vi "StatisticsGui.vi"() -> ()   [LabVIEW 2016]
uses:
  Logger/Logger.Stats.Fglb.Result.ctl
  StatisticsGui.Action.ctl
  Logger/Logger.Stats.Fglb.Action.ctl
  <vilib>/Utility/miscctls.llb/LVRowAndColumnTypeDef.ctl
  tools/CitTemplate/citTemplate.errData.ctl
  tools/EventLog/EventLog.EventSource.ctl
  tools/Config/Config.Global.vi
  Global/ApplicationGlobal.vi
  tools/Translator/Translator.Global.vi
  tools/Translator/Translator.Message.ctl
panel:
  out "Graph":cluster{"Graph":dbl[], "Graph":dbl[]}[](graph)
  out "MinTS":timestamp
  out "MaxTS":timestamp
  in  "Table/Graph":bool
  in  "Results.TimeTo":timestamp caption="To" format="%<%x %X>T"
  in  "Results.TimeFrom":timestamp caption="From" format="%<%x %X>T"
  in  "Text Ring":u16(ring) caption="Span"
  out "Results":T1[](array[typedef]) {"Time From" format="%<%X %x>T"; "Time To" format="%<%X %x>T"}
  in  "Values":i32[](listbox) caption="Data"
  out "ValuesRowSelected":i32
  in  "Hider":bool
  in  "StartHere...":bool
  out "_loop":i32(ring)=4
  out "Panel":refnum<vi>
  in  "ResultsAmount":i32=1 caption="Span" min=1 max=100
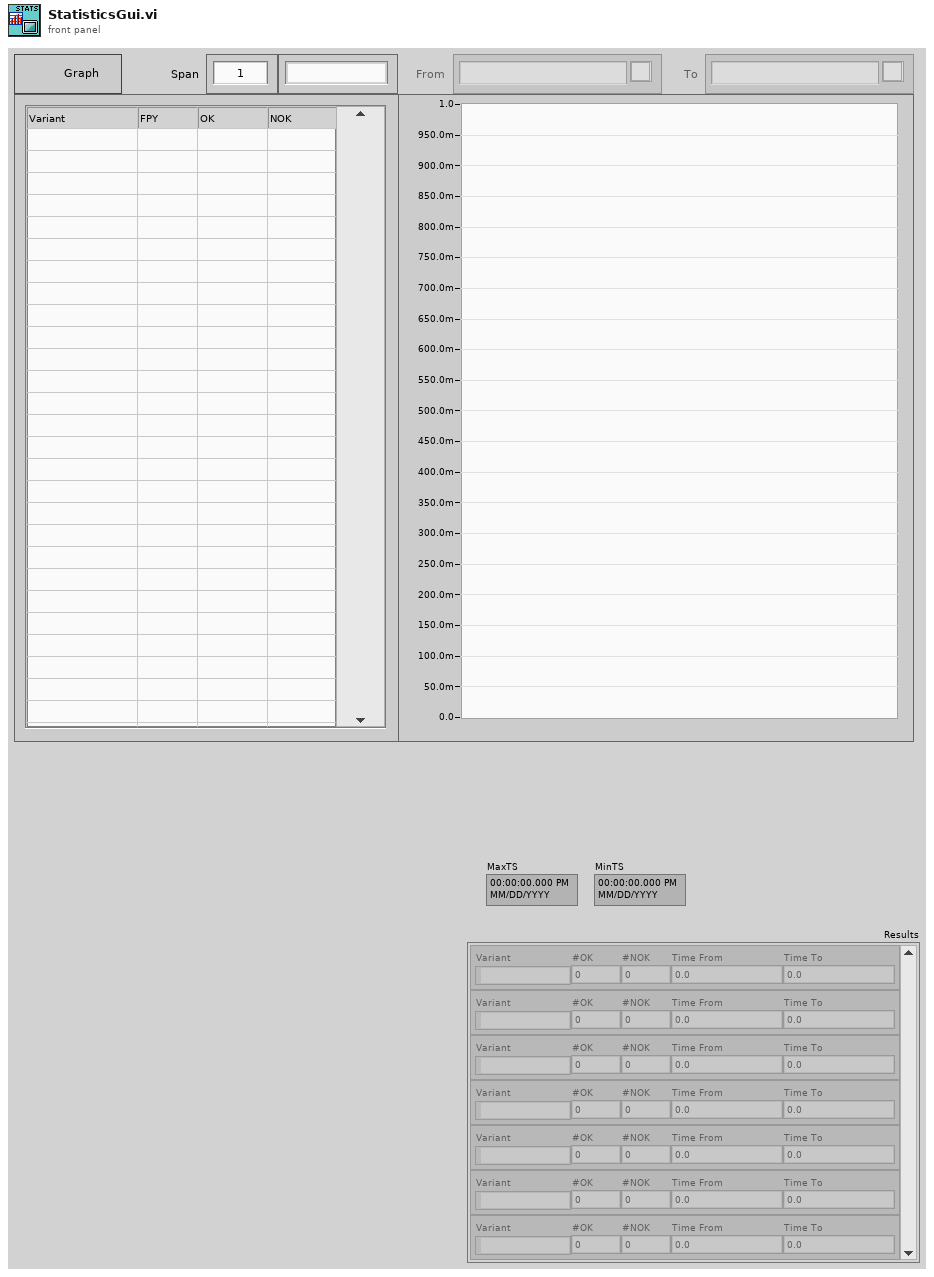
[diagram p1: front panel]
types:
  T1 = typedef "Logger.Stats.Fglb.Result.ctl" = cluster{"Variant":string, "#OK":i32, "#NOK":i32, "Time From":dbl, "Time To":dbl}
  T2 = typedef "StatisticsGui.Action.ctl" = enum32{"idle", "constructor", "destructor", "--- StatisticsGui ---", "new file", "update files", "update table", "update graph", "update time span"}
  T3 = enum8{"Enabled", "Disabled", "Disabled and Grayed Out"}
  T4 = typedef "Logger.Stats.Fglb.Action.ctl" = enum16{"init", "add", "get", "get all"}
  T5 = typedef "LVRowAndColumnTypeDef.ctl" = cluster{"Row":i32, "Column":i32}
  T6 = typedef "citTemplate.errData.ctl" = cluster{"ts":timestamp, "src":T7, "instance":i32, "action":string, "error":errorcluster, "unconfirmed":bool}
  T7 = typedef "EventLog.EventSource.ctl" = enum16{"All", "Gui", "Ref", "File", "Arch", "Seq", "CPX", "DB", "Laser", "Scan.P", "Scan.O"}
  T8 = typedef "citTemplate.notifierHandle.ctl" = refnum<notifier>
  T9 = enum32{"Invalid", "Standard", "Closed", "Hidden", "Minimized", "Maximized"}
  T10 = typedef "LVPoint32TypeDef.ctl" = cluster{"Horizontal":i32, "Vertical":i32}
  T11 = typedef "LVPositionTypeDef.ctl" = cluster{"Left":i32, "Top":i32}
  T12 = typedef "Translator.Message.ctl" = enum16{"-", "Event confirmed", "Log out", "Log in", "Shutdown", "Cancel", "Start", "Begin time", "End time", "Duration", "Service Mode", "Ignore Results", "Serial Format", "On", "Off", "OK", "NOK", "NOK %s", "Home", "Work", "Close", "Open", "In progress...", "Missing", "Empty", "Hardware failure", "Initial", "Default", "Total", "Out of range", "Free disk space is below 1GB - contact technician", "Error %d >> %s", "Error %d >> %s >> %s", "Msg %d >> %s", "Laser msg %d %s", "Laser cmd error %s %d", "Laser cmd failed %s", "Laser cmd warning %s", "Laser disconnected", "Laser status %s", "Laser already started", "Laser job unkonwn %s", "Laser job missing %s", "Laser job select failure %s", "Unable to start laser printing (%s)", "Unable to stop laser printing (%s)", "Laser marking aborted", "Laser marking timeout", "Unable to reset Laser Interlock (%s)", "Unable to trigger Laser. Laser not ready (%s)", "Laser job '%s' coordinates not configured", "Starting %s", "Quitting %s", "Configured", "Initializing", "Quitting", "Loading", "Loaded %d results", "Loaded %d events", "Running", "Stopped", "Summary", "Laser", "Do you want to continue?", "Do you want to delete the configuration?", "The configuration is being used by an order. Unable to delete!", "Press confirm button", "Station is not based. Do you want to exit?", "Station requires changeover. Do you want to run the test?", "Test options are not set as default. Do you want to continue?", "Formatting of WabcoNo is disabled. Do you want to continue?", "Product not detected. Do you want to continue?", "Product scan failed. Do you want to continue?", "Calibration", "Log out?", "System", "All", "IDLE", "Translating...%s", "Not found", "Alarm %s", "Run", "Skip", "Abort", "Repeat", "Please wait...", "Database disconnected", "Database disconnected - changeover disabled!", "Login to database successful", "Login to database failed: %d; %s", "Unable to check the product status of reference %d - database disconnected", "Unable to set the product status of reference %d - database disconnected", "Variant file backup %s", "Read variant (%s)", "Result", "Station armed!", "Station requires changeover!", "Select reference number...", "EMERGENCY BUTTON - press Control button", "EMERGENCY DOOR - press Control button", "Resetting Emergency...", "Unable to reset safety circuit - Emergency Button pressed", "Unable to reset safety circuit - Emergency Side Door open", "Station not based", "Station based", "Station not empty", "Station basing...", "No order", "Press Start to begin new order", "Scanning new order", "Order NOK. Correct or scan again", "Order OK. Press Accept", "Order ready", "Revolver incorrect", "Fork incorrect", "Revolver missing", "Revolver empty", "Container missing", "Offline results", "Offline statistics", "Updating statistics %.1f %%", "DMC Configurator", "Door open", "Close the front door", "Press start button", "Done. Open the front door", "Running...", "Running...%.1f %%", "Pause %s", "Pause %s. NOK container missing", "Pause %s. OK container missing", "Pause %s. Revolver empty", "Pause %s. Revolver missing", "Pause %s. Revolver incorrect", "Pause %s. Fork missing", "Pause %s. Fork incorrect", "Pause %s. Too many failures", "Pause %s. Unloading failure", "Pause %s. One slot is not working", "Pause %s. Part order is done. Empty OK container", "Pause %s. Unable to move product to slot", "Pause %s. Unable to move back product pusher", "Pause %s. Unable to lift product", "Pause %s. Unable to move back product lifter", "Pause %s. Unable to move product arm to Work", "Pause %s. Unable to move product arm to NOK", "Pause %s. Unable to move product arm to OK", "Pause %s. Unable to unsuck the NOK product", "Pause %s. Unable to drop the NOK product", "Pause %s. Product OK missing", "Pause %s. Unable to unsuck the OK product", "Pause %s. Unable to drop the OK product", "Stopping...", "File '%s' is missing", "File '%s' is broken", "File '%s' is running", "Log file started (%s)", "Log file ended (%s)", "Log file stopped (%s)", "Log file ignored (%s)", "Log file exported (%s)", "Log file export failed (%s)", "Wrong serial number in log file", "Wrong reference number in log file", "Test steps are missing", "%s = %.3f", "Process param '%s' not found in DB", "Process param '%s' wrong order", "Process param '%s' value %.3f out of limits (%.3f; %.3f)", "Step%d param '%s' not found in DB", "Step%d param '%s' wrong order", "Step%d param '%s' value %.3f out of limits (%.3f; %.3f)", "Step%d EV '%s' not found in DB", "Step%d EV '%s' wrong order", "\"%s\" not found in DB", "\"%s\" wrong order", "\"%s\" value %.3f out of limits (%.3f; %.3f)", "\"%s\" not found in software", "Process init (%s)", "Process started", "Process restarted", "Process run", "Process done", "Process done - remove OK container", "Process aborted", "Process aborted at work", "Process aborted at home", "Process error", "Process error at home", "Process error at work", "Process close", "Process pause", "Process continue", "Process door open", "Process door close", "Process pause at slot %s due to %s", "Select plate from the order to process", "Do you want to start the process?", "Do you want to continue the process?", "There is unfinished order. Do you want to put the new order?", "Product %s %d OK", "Product %s %d NOK", "Unable to unload the slot %s. Product missing in the slot", "Unable to unload the slot %s. Product already in the arm", "Unable to accept the product as OK. Product missing in slot %s", "Unable to accept the product as OK. Product could not drop into the container at slot %s", "Unable to accept the product as NOK. Product could not drop into the container at slot %s", "Scan failed. Error %s", "Scan failed. Scanner disconnected", "Scan failed. Wrong Wabco number %d, limit (%d,%d)", "Scan failed. Wrong serial number %d, limit (%d,%d)", "Scan failed. Wrong date %d, limit (%d,%d)", "Scan failed. Wrong product wabco number %d (expected %d)", "Scan failed. Wrong product serial number %d (expected > 0)", "Scan OK %s", "Scan failed. Unable to determine table position (%s)", "Scan failed. Timeout", "Tune failed. Scanner disconnected", "Tune failed. Timeout", "%s = %d", "%s = %d->%d", "Unable to set %s = %.2f - Air Pressure Inside off", "Unable to set digital output '%s' = %d", "Unable to activate air pressure inside - timeout", "Unable to activate air pressure inside - aborted", "Unable to switch on Air Main Valve - Air Pressure Inlet off", "Unable to switch on Air Main Valve - Door open", "Unable to switch off Air Main Valve - timeout", "Unable to switch off Air Main Valve - aborted", "Unable to rotate Table - timeout", "Unable to rotate Table - aborted", "Unable to rotate Table - Product Move not in Home position", "Unable to rotate Table - Air Pressure Inside off", "Unable to rotate Table - Product Lift A not in Home position", "Unable to rotate Table - Product Lift B not in Home position", "Unable to rotate Table - unlock before movement timeout", "Unable to rotate Table - lock after movement timeout", "Unable to move Table Lock to %s position - timeout", "Unable to move Table Lock to %s position - aborted", "Unable to move Table Lock to %s position - Air Pressure Inside off", "Unable to move Table Lock to %s position - Table not in position", "Unable to move Product Lift A to %s position - timeout", "Unable to move Product Lift B to %s position - timeout", "Unable to move Product Lift A to %s position - aborted", "Unable to move Product Lift B to %s position - aborted", "Unable to move Product Lift A to %s position - Air Pressure Inside off", "Unable to move Product Lift B to %s position - Air Pressure Inside off", "Unable to move Product Lift A to %s position - Table not locked", "Unable to move Product Lift B to %s position - Table not locked", "Unable to move Product Lift A to %s position - Product Arm not in Work position", "Unable to move Product Lift B to %s position - Product Arm not in Work position", "Unable to set Product Suction Gripper %s to %s - timeout", "Unable to set Product Suction Gripper %s to %s - aborted", "Unable to set Product Suction Gripper %s to %s - Air Pressure Inside off", "Unable to set Product Suction Gripper %s to %s - Table slot unkown", "Unable to move Product Arm to %s position - timeout", "Unable to move Product Arm to %s position - aborted", "Unable to move Product Arm to %s position - Air Pressure Inside off", "Unable to move Product Arm to %s position - Product Lift A not in Home position", "Unable to move Product Arm to %s position - Product Lift B not in Home position", "Unable to move Product to %s position - timeout", "Unable to move Product to %s position - aborted", "Unable to move Product to %s position - Air Pressure Inside off", "Unable to move Product to %s position - Table not in position"}
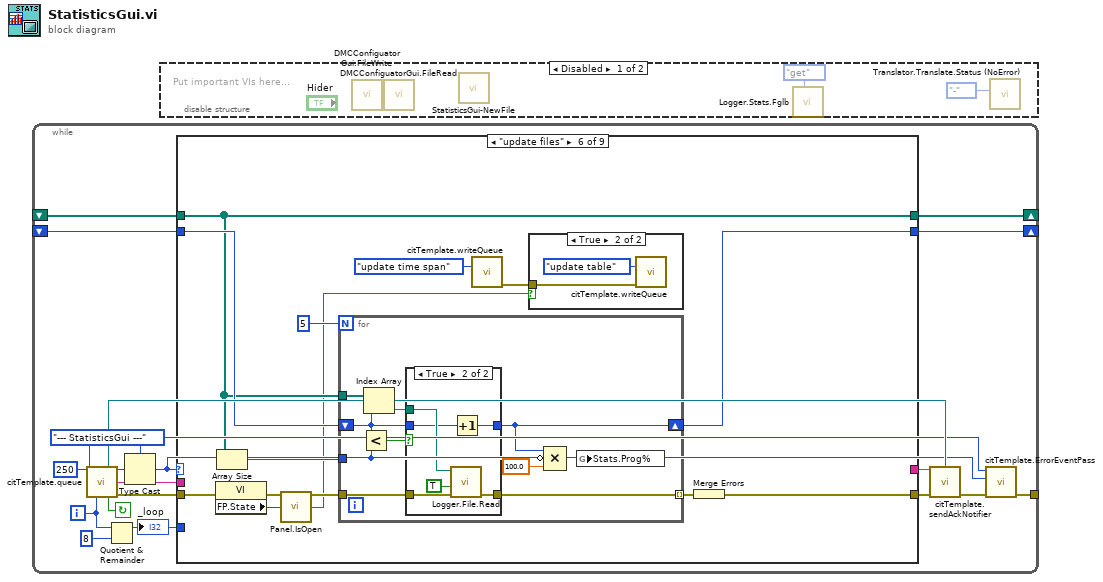
[diagram p0: block diagram]
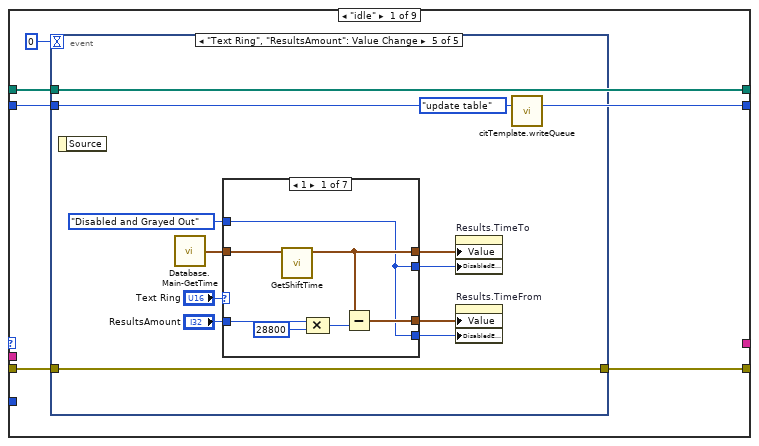
[diagram p2: hidden frame]
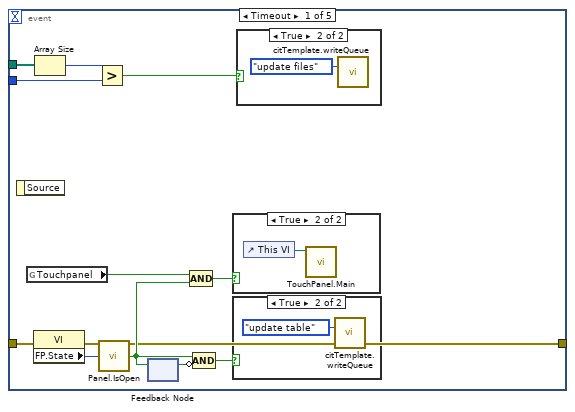
[diagram p3: hidden frame]
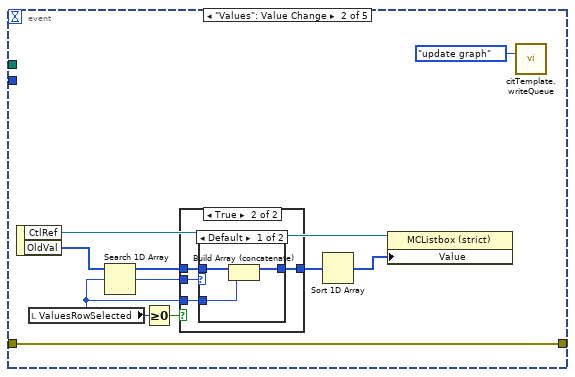
[diagram p7: hidden frame]
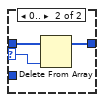
[diagram p9: hidden frame]
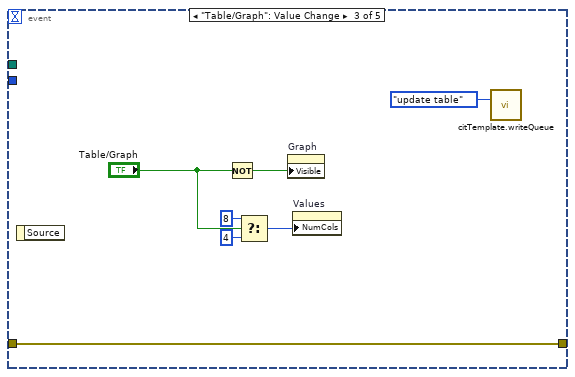
[diagram p10: hidden frame]
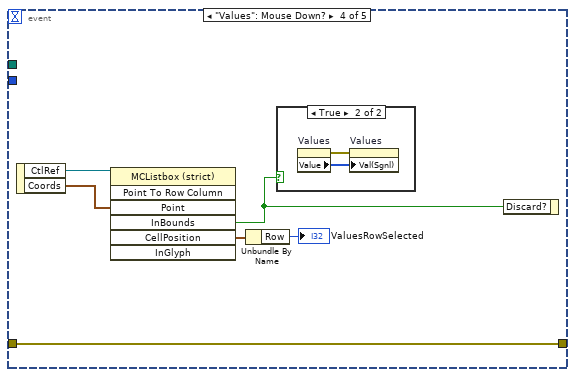
[diagram p11: hidden frame]
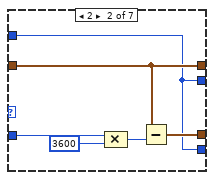
[diagram p13: hidden frame]
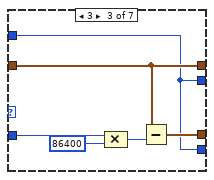
[diagram p14: hidden frame]
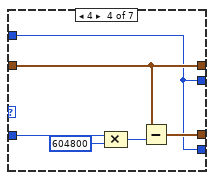
[diagram p15: hidden frame]
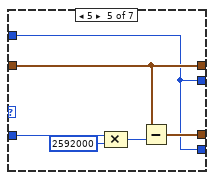
[diagram p16: hidden frame]
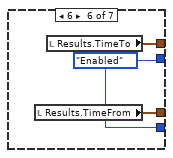
[diagram p17: hidden frame]
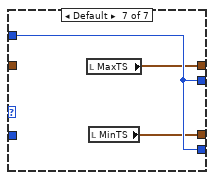
[diagram p18: hidden frame]
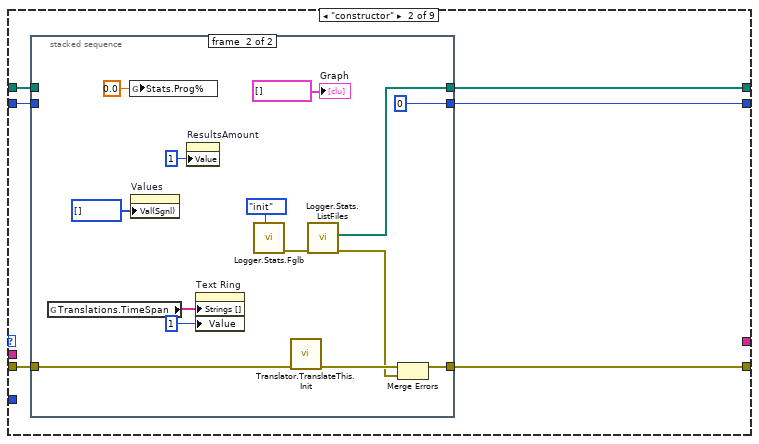
[diagram p19: hidden frame]
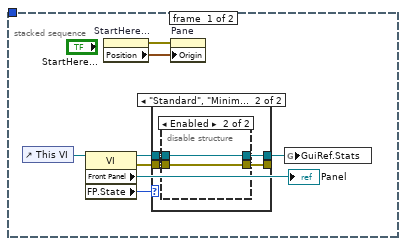
[diagram p20: hidden frame]
diagram:
  n1 = while {
    tunnel: [w7] -> _
    shift-right: [w4] -> _
    shift-left: _ -> [w3]
    shift-right: [w2] -> _
    shift-left: _ -> [w1]
    i -> [w9]
    stop <- w15 continue-if-true
    w12 = StatisticsGui.Action."--- StatisticsGui ---" ("Action")
    n2 = call "citTemplate.queue.vi"("ms timeout (250 ms)"=250, "event enum"=w12, "iteration (-1)"=w9) -> ("notifierHandle out"=w14:T8, "event out"=w18:u32, "(flatten) data out"=w17:string, "continue"=w15:bool, "error out"=w16:errorcluster)  [unwired: 2 in, 6 out]
    n3 = Quotient & Remainder(x=w9, y=8) -> (x-y*floor(x/y)=w5:i32)  [unwired: 1 out]
    "_loop" <- w5
    n4 = Type Cast(type=w12, x=w18) -> (*(type *) &x=w8:T2)
    n5 = case shown="\"update files\"" w8 {
      tunnel: w17 -> [_ _ _ w184 w193 _ _ _ _]
      tunnel: w16 -> [w23 w125 w163 w182 w192 w199 w230 w295 w319]
      tunnel: [_ _ _ "" _ _ _ _ _] -> w13
      tunnel: [w21 w126 w164 w183 w186 w196 w229 w296 w318] -> w11
      tunnel: w5 -> [_ _ _ _ _ _ _ _ _]
      tunnel: [w20 w124 w162 w178 w189 w203 w228 w294 w317] -> w4
      tunnel: w3 -> [w20 w123 w162 w178 w190 w203 w228 w294 w317]
      tunnel: [w19 w122 w161 w177 w191 w201 w227 w293 w316] -> w2
      tunnel: w1 -> [w19 w121 w161 w177 w191 w204 w227 w293 w316]
      frame "idle" {
        n6 = event shown="[4] \"Text Ring\", \"ResultsAmount\": Value Change" {
          selector: _ -> [_ _ _ _ _]
          dyn-events: _ -> [_ _ _ _ _]
          timeout: 0 -> [_ _ _ _ _]
          tunnel: w23 -> [w35 w45 w60 w66 w81]
          tunnel: [w24 w45 w60 w66 w81] -> w21
          tunnel: w20 -> [w28 _ _ _ _]
          tunnel: w19 -> [w26 _ _ _ _]
          event Timeout {
            n7 = event-data() -> ()  [unwired: 1 in, 1 out]
            n8 = global read "Config.Global.vi" "Touchpanel"() -> (w32:bool)
            n9 = property class="VI"(error in=w35) -> (error out=w24:errorcluster, "FP.State"=w33:T9)  [unwired: 1 in, 1 out]
            n10 = Array Size(array=w28) -> (size(s)=w25:i32)
            n11 = Greater?(x=w25, y=w26) -> (0:w27:bool)
            n12 = call "Panel.IsOpen.vi"("FP State"=w33) -> ("Open?"=w29:bool)
            n13 = feedback-in #1(w29) -> ()
            n14 = feedback #1() -> (w34:bool)  [unwired: 1 in]
            n15 = Compound Arithmetic op=AND(w32, w29) -> (w31:bool)
            n16 = Compound Arithmetic op=AND(w29, invert w34) -> (w30:bool)
            n17 = case shown="True" w31 {
              frame False {
              }
              frame True {
                n18 = control-ref of="This VI"() -> (w38:refnum<vi>)
                n19 = call "TouchPanel.Main.vi"("VI ref"=w38) -> ()  [unwired: 8 in, 3 out]
              }
            }
            n20 = case shown="True" w30 {
              frame False {
              }
              frame True {
                n21 = call "citTemplate.writeQueue.vi"("event in (if not connected:all statemachine with data event)"=StatisticsGui.Action."update table" ("Action")) -> ()  [unwired: 14 in, 1 out]
              }
            }
            n22 = case shown="True" w27 {
              frame False {
              }
              frame True {
                n23 = call "citTemplate.writeQueue.vi"("event in (if not connected:all statemachine with data event)"=StatisticsGui.Action."update files" ("Action")) -> ()  [unwired: 14 in, 1 out]
              }
            }
          }
          event "Values": Value Change {
            n24 = event-data() -> ("CtlRef"=w47:refnum<vi>, "OldVal"=w44:i32[])  [unwired: 1 in]
            n25 = local read "ValuesRowSelected"() -> (w41:i32)
            n26 = Search 1D Array(1D array=w44, element=w41) -> (index of element=w46:i32)  [unwired: 1 in]
            n27 = Greater Or Equal To 0?(x=w41) -> (x >= 0?=w43:bool)
            n28 = case shown="True" w43 {
              tunnel: w46 -> [_ w52]
              tunnel: w44 -> [w48 w51]
              tunnel: [w48 w50] -> w42
              tunnel: w41 -> [_ w49]
              frame False {
              }
              frame True {
                n29 = case shown="Default" w52 {
                  selector: w52 -> [_ w57]
                  tunnel: w51 -> [w55 w58]
                  tunnel: [w54 w56] -> w50
                  tunnel: w49 -> [w53 _]
                  frame Default {
                    n30 = Build Array (concatenate)(w55, w53) -> (w54:i32[])
                  }
                  frame 0.. {
                    n31 = Delete From Array(array=w58, index=w57) -> (array with subset deleted=w56:i32[])  [unwired: 1 in, 1 out]
                  }
                }
              }
            }
            n32 = Sort 1D Array(array=w42) -> (sorted array=w39:i32[])
            n33 = property class="MCListbox (strict)"(reference=w47, "Value"=w39) -> ()  [unwired: 1 in, 2 out]
            n34 = call "citTemplate.writeQueue.vi"("event in (if not connected:all statemachine with data event)"=StatisticsGui.Action."update graph" ("Action")) -> ()  [unwired: 14 in, 1 out]
          }
          event "Table/Graph": Value Change {
            n35 = event-data() -> ()  [unwired: 1 in, 1 out]
            n36 = Not(x="Table/Graph") -> (.not. x?=w65:bool)
            n37 = Select(t=u32 8 ("Number of Columns"), s="Table/Graph", f=u32 4 ("Number of Columns")) -> (s? t:f=w62:u32)
            n38 = property on="Graph" class="XYGraph (strict)"("Visible"=w65) -> ()  [unwired: 2 in, 2 out]
            n39 = property on="Values" class="MCListbox (strict)"("NumCols"=w62) -> ()  [unwired: 2 in, 2 out]
            n40 = call "citTemplate.writeQueue.vi"("event in (if not connected:all statemachine with data event)"=StatisticsGui.Action."update table" ("Action")) -> ()  [unwired: 14 in, 1 out]
          }
          event "Values": Mouse Down? {
            n41 = event-data() -> ("CtlRef"=w71:refnum<vi>, "Coords"=w70:T10)  [unwired: 1 in]
            n42 = invoke class="MCListbox (strict)" method="Point To Row Column"(reference=w71, "Point"=w70) -> ("InBounds"=w67:bool, "CellPosition"=w69:T5)  [unwired: 5 in, 5 out]
            n43 = Unbundle By Name(w69) -> ("Row"=→"ValuesRowSelected":i32)
            n44 = case shown="True" w67 {
              frame False {
              }
              frame True {
                n45 = property on="Values" class="MCListbox (strict)"() -> (error out=w73:errorcluster, "Value"=w72:i32[])  [unwired: 2 in, 1 out]
                n46 = property on="Values" class="MCListbox (strict)"(error in=w73, "Val(Sgnl)"=w72) -> ()  [unwired: 1 in, 2 out]
              }
            }
            n47 = event-data("Discard?"=w67) -> ()  [unwired: 1 in, 1 out]
          }
          event "Text Ring", "ResultsAmount": Value Change {
            n48 = event-data() -> ()  [unwired: 1 in, 1 out]
            n49 = call "Database.Main-GetTime.vi"() -> ("TS"=w74:timestamp)  [unwired: 1 in]
            n50 = case shown="1" "Text Ring" {
              tunnel: [w88 w95 w101 w107 w113 w117 w119] -> w80
              tunnel: w74 -> [w89 w95 w101 w107 w113 _ _]
              tunnel: [w85 w96 w102 w108 w114 w116 w118] -> w79
              tunnel: "ResultsAmount" -> [w87 w94 w100 w106 w112 _ _]
              tunnel: [w84 w91 w97 w103 w109 w115 w120] -> w78
              tunnel: [w84 w91 w97 w103 w109 w115 w120] -> w77
              tunnel: T3."Disabled and Grayed Out" ("Disabled") -> [w84 w91 w97 w103 w109 _ w120]
              frame 1 {
                n51 = call "GetShiftTime.vi"("Time"=w89) -> ("Shift End Time"=w88:timestamp)  [unwired: 7 in, 3 out]
                n52 = Compound Arithmetic op=MULTIPLY(w87, 28800) -> (w86:i32)
                n53 = Subtract(x=w88, y=w86) -> (x-y=w85:timestamp)
              }
              frame 2 {
                n54 = Compound Arithmetic op=MULTIPLY(w94, 3600) -> (w93:i32)
                n55 = Subtract(x=w95, y=w93) -> (x-y=w96:timestamp)
              }
              frame 3 {
                n56 = Compound Arithmetic op=MULTIPLY(w100, 86400) -> (w99:i32)
                n57 = Subtract(x=w101, y=w99) -> (x-y=w102:timestamp)
              }
              frame 4 {
                n58 = Compound Arithmetic op=MULTIPLY(w106, 604800) -> (w105:i32)
                n59 = Subtract(x=w107, y=w105) -> (x-y=w108:timestamp)
              }
              frame 5 {
                n60 = Compound Arithmetic op=MULTIPLY(w112, 2592000) -> (w111:i32)
                n61 = Subtract(x=w113, y=w111) -> (x-y=w114:timestamp)
              }
              frame 6 {
                w115 = T3."Enabled" ("Disabled")
                n62 = local read "Results.TimeFrom"() -> (w116:timestamp)
                n63 = local read "Results.TimeTo"() -> (w117:timestamp)
              }
              frame Default {
                n64 = local read "MaxTS"() -> (w119:timestamp)
                n65 = local read "MinTS"() -> (w118:timestamp)
              }
            }
            n66 = property on="Results.TimeTo" class="AbsTime (strict)"("Value"=w80, "DisabledEnum"=w77) -> ()  [unwired: 2 in, 2 out]
            n67 = property on="Results.TimeFrom" class="AbsTime (strict)"("Value"=w79, "DisabledEnum"=w78) -> ()  [unwired: 2 in, 2 out]
            n68 = call "citTemplate.writeQueue.vi"("event in (if not connected:all statemachine with data event)"=StatisticsGui.Action."update table" ("Action")) -> ()  [unwired: 14 in, 1 out]
          }
        }
      }
      frame "constructor" {
        n69 = stacked-sequence {
          tunnel: [_ w152] -> w126
          tunnel: w125 -> [_ w160]
          tunnel: [_ w158] -> w124
          tunnel: w123 -> [_ _]
          tunnel: [_ 0] -> w122
          tunnel: w121 -> [_ _]
          frame #0 {
            n70 = control-ref of="This VI"() -> (w132:refnum<vi>)
            n71 = property class="VI"(reference=w132) -> (reference out=w131:refnum<vi>, error out=w130:errorcluster, "Front Panel"=→"Panel":refnum<vi>, "FP.State"=w129:T9)  [unwired: 1 in]
            n72 = property on="StartHere..." class="Bool (strict)"() -> (error out=w134:errorcluster, "Position"=w133:T11)  [unwired: 2 in, 1 out]
            n73 = case shown="\"Standard\", \"Minimized\", \"Maximized\"" w129 {
              tunnel: w131 -> [w136 w140]
              tunnel: w130 -> [w135 w139]
              tunnel: [w136 w138] -> w128
              tunnel: [w135 w137] -> _
              frame Default {
              }
              frame "Standard", "Minimized", "Maximized" {
                n74 = disable-structure shown="Enabled" {
                  disable-tunnel: w140 -> [w144 w146]
                  disable-tunnel: w139 -> [w143 w145]
                  disable-tunnel: [w142 w146] -> w138
                  disable-tunnel: [w141 w145] -> w137
                  frame Disabled {
                    n75 = invoke class="VI" method="FP.Close"(reference=w144, error in=w143) -> (reference out=w142:refnum<vi>, error out=w141:errorcluster)  [unwired: 1 in, 1 out]
                  }
                  frame Enabled {
                  }
                }
              }
            }
            n76 = property on="Pane" class="Pane"(error in=w134, "Origin"=w133) -> ()  [unwired: 1 in, 2 out]
            n77 = global write "ApplicationGlobal.vi" "GuiRef.Stats"(w128) -> ()
          }
          frame #1 {
            n78 = global read "Translator.Global.vi" "Translations.TimeSpan"() -> (w149:string[])
            n79 = global write "ApplicationGlobal.vi" "Stats.Prog%"(0.0 ("Stats.Prog%")) -> ()
            n80 = property on="Values" class="MCListbox (strict)"("Val(Sgnl)"=i32[] [] ("Value (Signaling)")) -> ()  [unwired: 2 in, 2 out]
            n81 = property on="ResultsAmount" class="DigNum (strict)"("Value"=1 ("ResultsAmount")) -> ()  [unwired: 2 in, 2 out]
            n82 = property on="Text Ring" class="Ring (strict)"("Strings []"=w149, "Value"=1) -> ()  [unwired: 2 in, 2 out]
            n83 = call "Logger.Stats.Fglb.vi"("Action (get)"=Logger.Stats.Fglb.Action."init" ("Action")) -> ("error out"=w154:errorcluster)  [unwired: 9 in, 1 out]
            n84 = call "Translator.TranslateThis.Init.vi"("error in"=w160) -> ("error out"=w153:errorcluster)  [unwired: 10 in]
            n85 = call "Logger.Stats.ListFiles.vi"("error in (no error)"=w154) -> ("error out"=w151:errorcluster, "Files"=w158:path[])  [unwired: 9 in]
            n86 = Merge Errors(w153, w151) -> (w152:errorcluster)
            "Graph" <- cluster{"Graph":dbl[], "Graph":dbl[]}[] [] ("Graph")
          }
        }
      }
      frame "destructor" {
        n87 = stacked-sequence {
          tunnel: [_ w176] -> w164
          tunnel: w163 -> [_ w175]
          frame #0 {
            n88 = local read "Panel"() -> (w173:refnum<vi>)
            n89 = property class="Pnl"(reference=w173, "DeferPanUpdts"=FALSE ("Defer Panel Updates")) -> (reference out=w171:refnum<vi>, error out=w170:errorcluster)  [unwired: 1 in]
            n90 = Close Reference(reference=w171, error in (no error)=w170) -> ()  [unwired: 1 out]
            n91 = property on="Values" class="MCListbox (strict)"("ItemNames"=string[][] [] ("Item Names"), "ActiveCell"=T5 {"Row"=-2, "Column"=-2} ("Active Cell:Active Cell"), "CellBG"=u32 16448250, "ActiveCell"=T5 {"Row"=-1, "Column"=-2} ("Active Cell:Active Cell"), "CellBG"=u32 13816530) -> ()  [unwired: 2 in, 2 out]
          }
          frame #1 {
            n92 = property on="Text Ring" class="Ring (strict)"("Strings []"=string[] []) -> ()  [unwired: 2 in, 2 out]
            n93 = call "Translator.TranslateThis.Exit.vi"("error in"=w175) -> ("error out"=w176:errorcluster)  [unwired: 10 in]
          }
        }
      }
      frame "--- StatisticsGui ---" {
        n94 = Unflatten From String(type=T6 {"ts"=timestamp(0 s since 1904-01-01), "src"=enum."All", "instance"=0, "action"="", "error"={"status"=FALSE, "code"=0, "source"=""}, "unconfirmed"=FALSE} ("ErrData"), binary string=w184, error in (no error)=w182) -> (value=w180:T6)  [unwired: 4 out]
        n95 = Unbundle By Name(w180) -> ("error"=w179:errorcluster)
        n96 = call <vilib>:"Clear Errors.vi"("error in (no error)"=w179) -> ("error out"=w183:errorcluster)  [unwired: 5 in, 1 out]
      }
      frame "new file" {
        n97 = Unflatten From String(type=path "", binary string=w193, error in (no error)=w192) -> (value=w187:path, error out=w186:errorcluster)  [unwired: 3 out]
        n98 = Build Array (concatenate)(w190, w187) -> (w189:path[])
      }
      frame "update files" {
        n99 = property class="VI"(error in=w199) -> (error out=w198:errorcluster, "FP.State"=w200:T9)  [unwired: 1 in, 1 out]
        n100 = Array Size(array=w203) -> (size(s)=w202:i32)
        n101 = call "Panel.IsOpen.vi"("FP State"=w200) -> ("Open?"=w197:bool)
        n102 = for {
          N: 5 -> [_]
          tunnel: w203 -> [w216]
          shift-right: [w209] -> w201
          shift-left: w204 -> [w213]
          tunnel: w202 -> [w210]
          tunnel: w198 -> [w218]
          tunnel: [w217] -> w206 mode=indexing
          n103 = Less?(x=w213, y=w210) -> (x < y?=w214:bool)
          n104 = Index Array(array=w216, index=w213) -> (element=w215:path)
          n105 = case shown="True" w214 {
            tunnel: w218 -> [w220 w225]
            tunnel: [w220 w224] -> w217
            tunnel: [w219 w223] -> w209
            tunnel: w215 -> [_ w222]
            tunnel: w213 -> [w219 w221]
            frame False {
            }
            frame True {
              n106 = call "Logger.File.Read.vi"("error in (no error)"=w225, "Update Stats (F)"=TRUE, "file path"=w222) -> ("error out"=w224:errorcluster)  [unwired: 5 in, 3 out]
              n107 = Increment(x=w221) -> (x+1=w223:i32)
            }
          }
          n108 = Compound Arithmetic op=MULTIPLY(w209, invert w210, 100.0 ("value")) -> (w211:dbl)
          n109 = global write "ApplicationGlobal.vi" "Stats.Prog%"(w211) -> ()
        }
        n110 = call "citTemplate.writeQueue.vi"("event in (if not connected:all statemachine with data event)"=StatisticsGui.Action."update time span" ("Action")) -> ("error out"=w194:errorcluster)  [unwired: 14 in]
        n111 = case shown="True" w197 {
          tunnel: w194 -> [_ w207]
          frame False {
          }
          frame True {
            n112 = call "citTemplate.writeQueue.vi"("event in (if not connected:all statemachine with data event)"=StatisticsGui.Action."update table" ("Action"), "error in (no error)"=w207) -> ()  [unwired: 13 in, 1 out]
          }
        }
        n113 = Merge Errors(w206) -> (w196:errorcluster)
      }
      frame "update table" {
        n114 = stacked-sequence {
          seq-local: [_ w234 _ _ _] -> [_ _ _ w283 _]
          tunnel: w230 -> [_ _ w253 _ _]
          tunnel: [_ _ w252 _ _] -> w229
          frame #0 {
            n115 = local read "Panel"() -> (w231:refnum<vi>)
            n116 = property class="Pnl"(reference=w231, "DeferPanUpdts"=TRUE ("Defer Panel Updates")) -> ()  [unwired: 1 in, 2 out]
          }
          frame #1 {
            n117 = property on="Values" class="MCListbox (strict)"() -> (error out=w233:errorcluster, "ItemNames"=w236:string[][], "Value"=w235:i32[])  [unwired: 2 in, 1 out]
            n118 = for {
              tunnel: w236 -> [w244]
              tunnel: w235 -> [w243] mode=indexing
              tunnel: [w242] -> w234 mode=indexing
              n119 = Index Array(array=w244, index (row)=w243, index (col)=0 ("disabled index (col)")) -> (element=w242:string)
            }
            n120 = property on="Values" class="MCListbox (strict)"(error in=w233, "ActiveCell"=T5 {"Row"=-2, "Column"=-2} ("Active Cell:Active Cell"), "CellBG"=u32 16448250, "ActiveCell"=T5 {"Row"=-1, "Column"=-2} ("Active Cell:Active Cell"), "CellBG"=u32 13816530) -> ()  [unwired: 1 in, 2 out]
          }
          frame #2 {
            n121 = To Double Precision Float(number="Results.TimeFrom") -> (double precision float=w246:dbl)
            n122 = To Double Precision Float(number="Results.TimeTo") -> (double precision float=w248:dbl)
            n123 = call "Logger.Stats.Fglb.vi"("Time To"=w248, "Time From"=w246, "Action (get)"=Logger.Stats.Fglb.Action."get" ("Action"), "error in (no error)"=w253) -> ("error out"=w252:errorcluster, "Results"=w250:T1[])  [unwired: 6 in]
            "Results" <- w250
            n124 = call "citTemplate.writeQueue.vi"("event in (if not connected:all statemachine with data event)"=StatisticsGui.Action."update graph" ("Action")) -> ()  [unwired: 14 in, 1 out]
            n125 = for {
              tunnel: w250 -> [w269] mode=indexing
              tunnel: [w281] -> w251 mode=indexing
              i -> [w264]
              w278 = "%Y-%m-%d %H:%M:%S" ("time format string (%c)")
              n126 = Unbundle(w269) -> ("Variant"=w257:string, "#OK"=w267:i32, "#NOK"=w268:i32, "Time From"=w256:dbl, "Time To"=w255:dbl)
              n127 = Compound Arithmetic op=ADD(w267, w268) -> (w261:i32)
              n128 = Bundle(w264, "precision (6)"=i16 1) -> (w262:cluster{i32, "precision (6)":i16})  [unwired: 1 in]
              n129 = call "Int2Str.vi"("Numeric"=w267) -> ("string"=w280:string)
              n130 = Compound Arithmetic op=MULTIPLY(100.0 ("value"), w267, invert w261) -> (w259:dbl)
              n131 = call "Int2Str.vi"("Numeric"=w268) -> ("string"=w279:string)
              n132 = call "DblNaN2Str.vi"("Numeric"=w259, "precision (6)"=i16 2) -> ("string"=w266:string)
              n133 = Format Date/Time String(time format string (%c)=w278, seconds (now)=w256) -> (date/time string=w277:string)  [unwired: 1 in]
              n134 = Format Date/Time String(time format string (%c)=w278, seconds (now)=w255) -> (date/time string=w275:string)  [unwired: 1 in]
              n135 = Greater Than 0?(x=w256) -> (x > 0?=w276:bool)
              n136 = Greater Than 0?(x=w255) -> (x > 0?=w274:bool)
              n137 = call "StatisticsGui.FPYcolor.vi"("result"=w259) -> ("Color"=w258:u32)
              n138 = Select(t=w277, s=w276, f="") -> (s? t:f=w271:string)
              n139 = Select(t=w275, s=w274, f="") -> (s? t:f=w270:string)
              n140 = property on="Values" class="MCListbox (strict)"("ActiveCell"=w262, "CellBG"=w258) -> ()  [unwired: 2 in, 2 out]
              n141 = Build Array(w257, w266, w280, w279, w271, w270) -> (w281:string[])
            }
            n142 = property on="Values" class="MCListbox (strict)"("ItemNames"=w251) -> ()  [unwired: 2 in, 2 out]
          }
          frame #3 {
            n143 = property on="Values" class="MCListbox (strict)" props=["ItemNames", "Value"]() -> ("ItemNames"=w286:string[][])  [unwired: 2 in, 3 out]
            n144 = Index Array(array=w286, index (col)=0 ("disabled index (col)")) -> (element=w284:string[])  [unwired: 1 in]
            n145 = for {
              tunnel: w284 -> [w290]
              tunnel: w283 -> [w289] mode=indexing
              tunnel: [w288] -> w282 mode=indexing if=w287
              n146 = Search 1D Array(1D array=w290, element=w289) -> (index of element=w288:i32)  [unwired: 1 in]
              n147 = Greater Or Equal To 0?(x=w288) -> (x >= 0?=w287:bool)
            }
            n148 = property on="Values" class="MCListbox (strict)"("Value"=w282) -> ()  [unwired: 2 in, 2 out]
          }
          frame #4 {
            n149 = local read "Panel"() -> (w291:refnum<vi>)
            n150 = property class="Pnl"(reference=w291, "DeferPanUpdts"=FALSE ("Defer Panel Updates")) -> ()  [unwired: 1 in, 2 out]
          }
        }
      }
      frame "update graph" {
        n151 = stacked-sequence {
          tunnel: [_ w302 _] -> w296
          tunnel: w295 -> [_ w301 _]
          frame #0 {
            n152 = local read "Panel"() -> (w297:refnum<vi>)
            n153 = property class="Pnl"(reference=w297, "DeferPanUpdts"=TRUE ("Defer Panel Updates")) -> ()  [unwired: 1 in, 2 out]
          }
          frame #1 {
            n154 = control-ref of="Graph"() -> (w299:refnum<vi>)
            n155 = local read "Results"() -> (w303:T1[])
            n156 = call "Logger.Stats.UpdateGraph.vi"("error in (no error)"=w301, "Selection"="Values", "Results"=w303, "Graph"=w299) -> ("error out"=w302:errorcluster)  [unwired: 7 in]
          }
          frame #2 {
            n157 = local read "Panel"() -> (w304:refnum<vi>)
            n158 = property class="Pnl"(reference=w304, "DeferPanUpdts"=FALSE ("Defer Panel Updates")) -> ()  [unwired: 1 in, 2 out]
          }
        }
      }
      frame "update time span" {
        n159 = call "Logger.Stats.Fglb.vi"("Action (get)"=Logger.Stats.Fglb.Action."get all" ("Action"), "error in (no error)"=w319) -> ("error out"=w318:errorcluster, "Results"=w315:T1[])  [unwired: 8 in]
        n160 = for {
          tunnel: w315 -> [w323] mode=indexing
          tunnel: [w322] -> w314 mode=indexing
          tunnel: [w321] -> w313 mode=indexing
          n161 = Unbundle(w323) -> ("Time From"=w322:dbl, "Time To"=w321:dbl)  [unwired: 3 out]
        }
        n162 = Build Array (concatenate)(w314, w313) -> (w312:dbl[])
        n163 = Array Max & Min(array=w312) -> (max value=w311:dbl, min value=w308:dbl)  [unwired: 2 out]
        n164 = To Time Stamp(1:w311) -> (0:→"MaxTS":timestamp)
        n165 = To Time Stamp(1:w308) -> (0:→"MinTS":timestamp)
        n166 = property on="Text Ring" class="Ring (strict)"() -> (error out=w307:errorcluster, "Value"=w306:u16)  [unwired: 2 in, 1 out]
        n167 = property on="Text Ring" class="Ring (strict)"(error in=w307, "Val(Sgnl)"=w306) -> ()  [unwired: 1 in, 2 out]
      }
    }
    n168 = call "citTemplate.sendAckNotifier.vi"("notification data"=w13, "notifierHandle in"=w14, "error in"=w11) -> ()  [unwired: 13 out]
    n169 = call "citTemplate.ErrorEventPass.vi"("error in"=w11, "action of error"=w8, "event in"=w12) -> ("error out"=w7:errorcluster)  [unwired: 2 in, 6 out]
  }
  n170 = disable-structure shown="Disabled" {
    frame Disabled {
      # "Put important VIs here..."
      n171 = call "DMCConfiguatorGui.FileWrite.vi"() -> ()  [unwired: 11 in, 1 out]
      n172 = call "DMCConfiguatorGui.FileRead.vi"() -> ()  [unwired: 10 in, 2 out]
      n173 = call "StatisticsGui-NewFile.vi"() -> ()  [unwired: 11 in, 1 out]
      n174 = call "Logger.Stats.Fglb.vi"("Action (get)"=Logger.Stats.Fglb.Action."get" ("Action")) -> ()  [unwired: 9 in, 2 out]
      n175 = call "Translator.Translate.Status (NoError).vi"("msg"=Translator.Message."-") -> ()  [unwired: 10 in, 1 out]
    }
    frame Enabled {
    }
  }
